vi "五参数标样核查.vi"(11 "启动参数":T1={"测量模式"="标样核查", "数据类型"="N", "输出参数"={"水温"=FALSE, "pH"=FALSE, "DO"=FALSE, "浊度"=FALSE, "电导率"=FALSE, "叶绿素a"=FALSE, "蓝绿藻"=FALSE, "藻密度"=FALSE, "ORP"=FALSE}}) -> ()   [LabVIEW 2016, in "斯坦道原位多参数.lvlib"]
panel:
  out "枚举":T2(ring)
  out "状态":string
  out "数值":i32
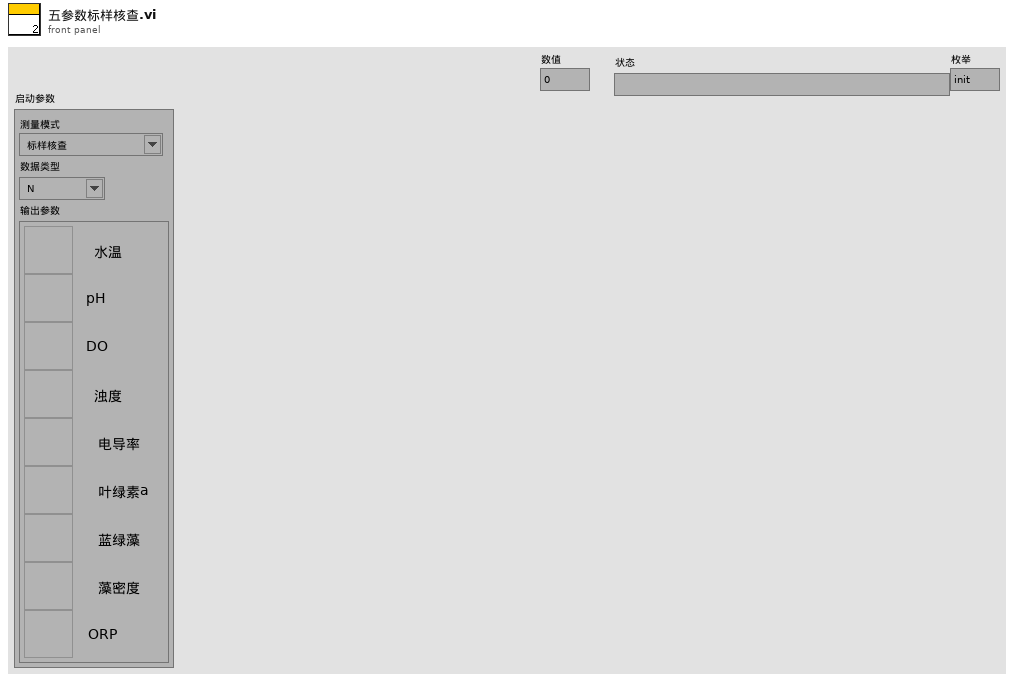
[diagram p1: front panel]
types:
  T1 = typedef "斯坦道原位多参数.lvlib/标样核查启动自定义输入参数.ctl" = cluster{"测量模式":string, "数据类型":string, "输出参数":cluster{"水温":bool, "pH":bool, "DO":bool, "浊度":bool, "电导率":bool, "叶绿素a":bool, "蓝绿藻":bool, "藻密度":bool, "ORP":bool}}
  T2 = enum16{"init", "开机", "启动测量", "读取测量值", "存储数据", "关闭测量", "关机", "结束"}
  T3 = cluster{"时间标识":timestamp, "设备":string, "日志信息":string, "流程参数":string}
  T4 = cluster{"系统时间":timestamp, "工作状态":u16, "测量模式":u16, "告警代码":enum16{"无告警", "缺试剂告警", "缺水样告警", "缺蒸馏水告警", "缺标液告警", "仪表漏液告警", "标定异常告警", "超量程告警", "加热异常", "低试剂预警", "超上限告警", "超下限告警", "仪表内部其他异常", "滴定异常告警", "电极异常告警", "量程切换告警", "参数设置告警", "PH电极电位异常", "电导率电极异常", "浊度光度异常", "溶解氧电极异常", "溶解氧光强异常", "温度异常告警", "PH异常告警", "溶解氧异常告警", "电导率异常告警", "浊度异常告警", "叶绿素异常告警", "藻密度异常告警", "蓝绿藻异常告警", "ORP异常告警", "氨氮异常告警", "清洁刷异常告警", "SD卡异常告警", "蓝牙异常告警", "Wifi异常告警", "流程异常告警"}, "故障代码":enum16{"无故障", "电机故障", "温度故障", "通讯故障", "滴定故障"}, "日志代码":u16, "软件版本":string}
  T5 = cluster{"水温标准液标准浓度":dbl, "酸碱度标准液标准浓度":dbl, "溶解氧标准液标准浓度":dbl, "电导率标准液标准浓度":dbl, "浊度标准液标准浓度":dbl, "叶绿素a标准液标准浓度":dbl, "蓝绿藻标准液标准浓度":dbl, "ORP标准液标准浓度":dbl, "藻密度标准液标准浓度":dbl}
  T6 = cluster{"因子编码":string, "单位":string, "标样参考值":sgl, "水样数据时间":timestamp, "水样实测值":sgl, "水样数据标识":string, "K":sgl, "B":sgl, "T":sgl, "H":sgl, "水深":sgl, "探头温度":sgl, "信号值":sgl}
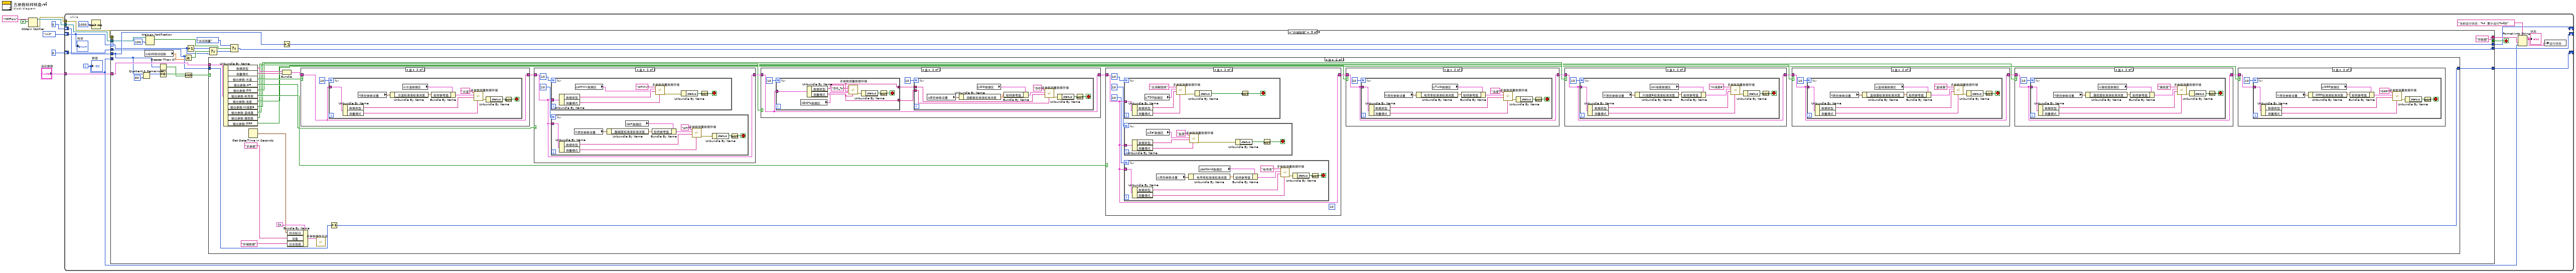
[diagram p0: block diagram]
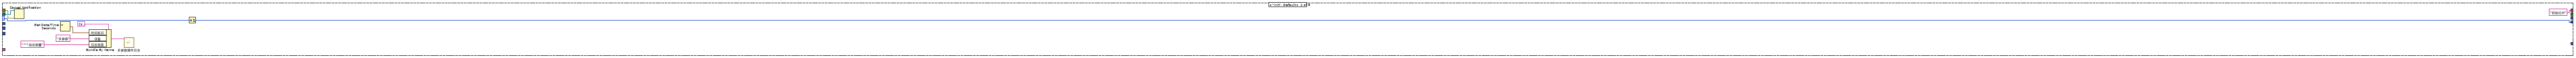
[diagram p2: hidden frame]
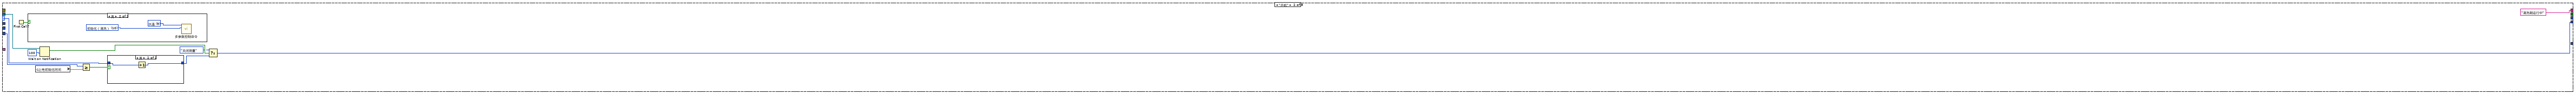
[diagram p3: hidden frame]
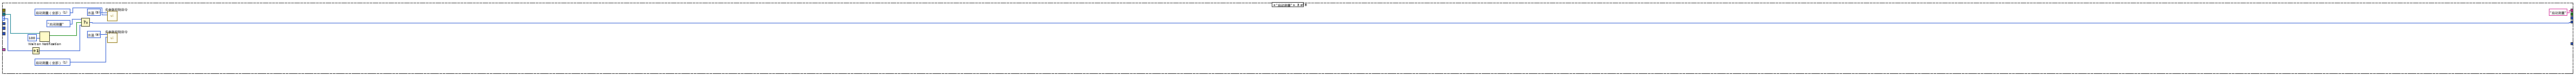
[diagram p6: hidden frame]
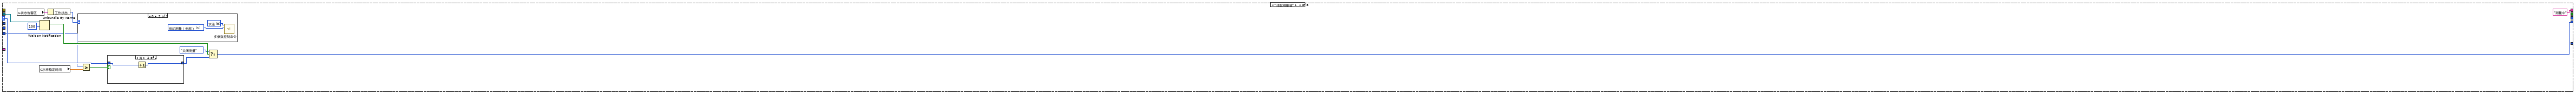
[diagram p7: hidden frame]
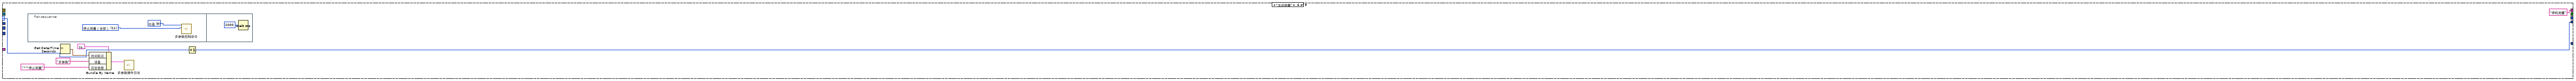
[diagram p20: hidden frame]
diagram:
  n1 = Obtain Notifier(name (unnamed)="MPFlow" ("名称（未命名）"), notification data type=FALSE) -> (notifier out=w5:refnum<notifier>, error out=w4:errorcluster)  [unwired: 2 in, 1 out]
  n2 = while {
    shift-right: [w19] -> _
    shift-left: T2."init" ("枚举") -> [w23]
    tunnel: w5 -> [w21]
    tunnel: w4 -> [w20]
    tunnel: "启动参数" -> [w13]
    shift-right: [w11] -> _
    shift-left: u32 0 ("等待时间（毫秒）") -> [w12]
    shift-right: [w9] -> _
    shift-left: u32 0 ("等待时间（毫秒）") -> [w10]
    i -> [w15]
    stop <- w22 stop-if-true
    n3 = Wait (ms)(milliseconds to wait=u32 1000 ("等待时间（毫秒）")) -> ()  [unwired: 1 out]
    n4 = case shown="\"存储数据\"" w23 {
      selector: w23 -> [w31 w45 w62 w75 w82 w300 w306 w310]
      tunnel: [_ _ _ _ _ _ _ TRUE] -> w22
      tunnel: w21 -> [w33 w41 w61 w72 w91 _ _ w307]
      tunnel: w20 -> [w32 _ _ _ _ _ _ _]
      tunnel: [w30 w39 w58 w70 w87 w299 w305 w309] -> w19
      tunnel: w15 -> [_ w44 _ w66 _ _ _ _]
      tunnel: ["初始化中" ("状态") "清洗刷运行中" ("状态") "启动测量" ("状态") "测量中" ("状态") "存数据" ("状态") "停机测量" ("状态") "关机" ("状态") "" ("状态")] -> w16
      tunnel: w13 -> [_ _ _ _ w100 _ _ _]
      tunnel: w12 -> [_ _ _ _ w94 _ _ _]
      tunnel: [_ _ _ _ w95 _ _ _] -> w11
      tunnel: w10 -> [_ _ _ _ w84 _ _ _]
      tunnel: [_ _ _ _ w86 _ _ _] -> w9
      frame "init", Default {
        n5 = Cancel Notification(0:w33, 3:w32) -> ()  [unwired: 3 out]
        n6 = Get Date/Time In Seconds() -> (seconds since 1Jan1904=w27:timestamp)
        n7 = Bundle By Name(cluster=T3 {"时间标识"=timestamp(0 s since 1904-01-01), "设备"="", "日志信息"="", "流程参数"=""} ("data in"), "时间标识"=w27, "设备"="多参数", "日志信息"="<<启动测量") -> (w26:T3)
        n8 = call "多参数操作日志.vi"("data"=w26) -> ()  [unwired: 10 in, 1 out]
        n9 = Increment(x=w31) -> (x+1=w30:T2)
      }
      frame "开机" {
        n10 = First Call?() -> (First Call?: T/F=w35:bool)
        n11 = case shown="真" w35 {
          frame False {
          }
          frame True {
            w47 = u16 10 items=["启动测量（全部）"=1, "初始化（清洗）"=10, "停止测量（全部）"=11, "校时"=13, "启动测量（单个传感器）"=19, "停止测量（单个传感器）"=20] ("控制命令")
            w46 = u16 9 items=["氨氮"=3, "水温"=9, "pH值"=10, "溶解氧"=11, "电导率"=12, "浊度"=13, "叶绿素a"=14, "藻密度"=15, "蓝绿藻"=16, "氧化还原电位"=17, "溶解氧%"=18, "盐度"=19] ("站号")
            n12 = call "多参数控制命令.vi"("控制命令"=w47, "站号"=w46) -> ()  [unwired: 9 in, 1 out]
          }
        }
        n13 = global read "多参数断电保存全局变量.vi" "上电初始化时间"() -> (w34:dbl)
        n14 = Wait on Notification(notifier=w41, timeout in ms (-1)=100 ("超时毫秒(-1)")) -> (notification=w42:bool)  [unwired: 2 in, 3 out]
        n15 = Greater Or Equal?(x=w44, y=w34) -> (x >= y?=w43:bool)
        n16 = case shown="真" w43 {
          tunnel: w45 -> [w48 w50]
          tunnel: [w48 w49] -> w40
          frame False {
          }
          frame True {
            n17 = Increment(x=w50) -> (x+1=w49:T2)
          }
        }
        n18 = Select(t=T2."关闭测量" ("枚举"), s=w42, f=w40) -> (s? t:f=w39:T2)
      }
      frame "启动测量" {
        w52 = u16 1 items=["启动测量（全部）"=1, "初始化（清洗）"=10, "停止测量（全部）"=11, "校时"=13, "启动测量（单个传感器）"=19, "停止测量（单个传感器）"=20] ("控制命令")
        w51 = u16 9 items=["氨氮"=3, "水温"=9, "pH值"=10, "溶解氧"=11, "电导率"=12, "浊度"=13, "叶绿素a"=14, "藻密度"=15, "蓝绿藻"=16, "氧化还原电位"=17, "溶解氧%"=18, "盐度"=19] ("站号")
        w53 = u16 1 items=["启动测量（全部）"=1, "初始化（清洗）"=10, "停止测量（全部）"=11, "校时"=13, "启动测量（单个传感器）"=19, "停止测量（单个传感器）"=20] ("控制命令")
        w54 = u16 9 items=["氨氮"=3, "水温"=9, "pH值"=10, "溶解氧"=11, "电导率"=12, "浊度"=13, "叶绿素a"=14, "藻密度"=15, "蓝绿藻"=16, "氧化还原电位"=17, "溶解氧%"=18, "盐度"=19] ("站号")
        n19 = Increment(x=w62) -> (x+1=w59:T2)
        n20 = Wait on Notification(notifier=w61, timeout in ms (-1)=100 ("超时毫秒(-1)")) -> (notification=w60:bool)  [unwired: 2 in, 3 out]
        n21 = Select(t=T2."关闭测量" ("枚举"), s=w60, f=w59) -> (s? t:f=w58:T2)
        n22 = call "多参数控制命令.vi"("控制命令"=w53, "站号"=w54) -> ()  [unwired: 9 in, 1 out]
        n23 = call "多参数控制命令.vi"("控制命令"=w52, "站号"=w51) -> ()  [unwired: 9 in, 1 out]
      }
      frame "读取测量值" {
        n24 = global read "多参数全局变量.vi" "状态告警区"() -> (w65:T4)
        n25 = global read "多参数断电保存全局变量.vi" "水样稳定时间"() -> (w63:dbl)
        n26 = Wait on Notification(notifier=w72, timeout in ms (-1)=100 ("超时毫秒(-1)")) -> (notification=w73:bool)  [unwired: 2 in, 3 out]
        n27 = Unbundle By Name(w65) -> ("工作状态"=w64:u16)
        n28 = case shown="0" w64 {
          frame Default {
          }
          frame 0 {
            w76 = u16 1 items=["启动测量（全部）"=1, "初始化（清洗）"=10, "停止测量（全部）"=11, "校时"=13, "启动测量（单个传感器）"=19, "停止测量（单个传感器）"=20] ("控制命令")
            w77 = u16 9 items=["氨氮"=3, "水温"=9, "pH值"=10, "溶解氧"=11, "电导率"=12, "浊度"=13, "叶绿素a"=14, "藻密度"=15, "蓝绿藻"=16, "氧化还原电位"=17, "溶解氧%"=18, "盐度"=19] ("站号")
            n29 = call "多参数控制命令.vi"("控制命令"=w76, "站号"=w77) -> ()  [unwired: 9 in, 1 out]
          }
        }
        n30 = Greater Or Equal?(x=w66, y=w63) -> (x >= y?=w74:bool)
        n31 = case shown="真" w74 {
          tunnel: w75 -> [w78 w80]
          tunnel: [w78 w79] -> w71
          frame False {
          }
          frame True {
            n32 = Increment(x=w80) -> (x+1=w79:T2)
          }
        }
        n33 = Select(t=T2."关闭测量" ("枚举"), s=w73, f=w71) -> (s? t:f=w70:T2)
      }
      frame "存储数据" {
        n34 = Quotient & Remainder(x=w94, y=u32 60) -> (x-y*floor(x/y)=w98:u32)  [unwired: 1 out]
        n35 = global read "多参数断电保存全局变量.vi" "标样测试组数"() -> (w81:dbl)
        n36 = Wait on Notification(notifier=w91, timeout in ms (-1)=100 ("超时毫秒(-1)")) -> (notification=w90:bool)  [unwired: 2 in, 3 out]
        n37 = Greater Than 0?(x=w94) -> (x > 0?=w93:bool)
        n38 = Equal To 0?(x=w98) -> (x = 0?=w97:bool)
        n39 = Greater Or Equal?(x=w84, y=w81) -> (x >= y?=w85:bool)
        n40 = Compound Arithmetic op=AND ("复合运算")(w97, w93) -> (w96:bool)
        n41 = Increment(x=w82) -> (x+1=w83:T2)
        n42 = Select(t=w83, s=w85, f=w82) -> (s? t:f=w89:T2)
        n43 = case shown="真" w96 {
          tunnel: w100 -> [_ w130]
          tunnel: w84 -> [w102 w112]
          tunnel: [w102 w111] -> w86
          frame False {
          }
          frame True {
            n44 = Unbundle By Name(w130) -> ("数据类型"=w129:string, "测量模式"=w128:string, "输出参数.水温"=w117:bool, "输出参数.pH"=w116:bool, "输出参数.DO"=w115:bool, "输出参数.电导率"=w114:bool, "输出参数.浊度"=w113:bool, "输出参数.叶绿素a"=w106:bool, "输出参数.蓝绿藻"=w105:bool, "输出参数.藻密度"=w104:bool, "输出参数.ORP"=w103:bool)
            n45 = Get Date/Time In Seconds() -> (seconds since 1Jan1904=w121:timestamp)
            n46 = Bundle("数据类型"=w129, "测量模式"=w128) -> (w127:cluster{"数据类型":string, "测量模式":string})  [unwired: 1 in]
            n47 = Bundle By Name(cluster=T3 {"时间标识"=timestamp(0 s since 1904-01-01), "设备"="", "日志信息"="", "流程参数"=""} ("data in"), "时间标识"=w121, "设备"="多参数", "日志信息"="存储数据") -> (w120:T3)
            n48 = case shown="真" w117 {
              tunnel: w127 -> [w279 w281]
              tunnel: [w279 w281] -> w126
              frame False {
              }
              frame True {
                n49 = for {
                  N: 10 -> [_]
                  tunnel: w281 -> [w292]
                  stop <- w286 stop-if-true
                  n50 = Unbundle By Name(w292) -> ("数据类型"=w283:string, "测量模式"=w282:string)
                  n51 = global read "多参数断电保存全局变量.vi" "质控参数设置"() -> (w290:T5)
                  n52 = Unbundle By Name(w290) -> ("水温标准液标准浓度"=w289:dbl)
                  n53 = global read "多参数全局变量.vi" "水温数据区"() -> (w291:T6)
                  n54 = Bundle By Name(cluster=w291, "标样参考值"=w289) -> (w285:T6)
                  n55 = call "多参数测量数据存储.vi"("测量模式"=w282, "数据类型"=w283, "数据区"=w285, "table输入"="水温") -> ("error out"=w288:errorcluster)  [unwired: 7 in]
                  n56 = Unbundle By Name(w288) -> ("status"=w287:bool)
                  n57 = Not(x=w287) -> (.not. x?=w286:bool)
                }
              }
            }
            n58 = call "多参数操作日志.vi"("data"=w120) -> ()  [unwired: 10 in, 1 out]
            n59 = Increment(x=w112) -> (x+1=w111:u32)
            n60 = case shown="真" w116 {
              tunnel: w126 -> [w256 w259]
              tunnel: [w256 w259] -> w124
              frame False {
              }
              frame True {
                n61 = for {
                  N: 10 -> [_]
                  tunnel: w259 -> [w267]
                  stop <- w264 stop-if-true
                  n62 = Unbundle By Name(w267) -> ("数据类型"=w261:string, "测量模式"=w260:string)
                  n63 = global read "多参数全局变量.vi" "pHmv数据区"() -> (w262:T6)
                  n64 = call "多参数测量数据存储.vi"("测量模式"=w260, "数据类型"=w261, "数据区"=w262, "table输入"="pHmv") -> ("error out"=w266:errorcluster)  [unwired: 7 in]
                  n65 = Unbundle By Name(w266) -> ("status"=w265:bool)
                  n66 = Not(x=w265) -> (.not. x?=w264:bool)
                }
                n67 = for {
                  N: 10 -> [_]
                  tunnel: w259 -> [w278]
                  stop <- w272 stop-if-true
                  n68 = Unbundle By Name(w278) -> ("数据类型"=w269:string, "测量模式"=w268:string)
                  n69 = global read "多参数断电保存全局变量.vi" "质控参数设置"() -> (w277:T5)
                  n70 = Unbundle By Name(w277) -> ("酸碱度标准液标准浓度"=w276:dbl)
                  n71 = global read "多参数全局变量.vi" "pH数据区"() -> (w275:T6)
                  n72 = Bundle By Name(cluster=w275, "标样参考值"=w276) -> (w270:T6)
                  n73 = call "多参数测量数据存储.vi"("测量模式"=w268, "数据类型"=w269, "数据区"=w270, "table输入"="pH") -> ("error out"=w274:errorcluster)  [unwired: 7 in]
                  n74 = Unbundle By Name(w274) -> ("status"=w273:bool)
                  n75 = Not(x=w273) -> (.not. x?=w272:bool)
                }
              }
            }
            n76 = case shown="真" w115 {
              tunnel: [w232 w237] -> w125
              tunnel: w124 -> [w232 w237]
              frame False {
              }
              frame True {
                n77 = for {
                  N: 10 -> [_]
                  tunnel: w237 -> [w255]
                  tunnel: [w249] -> w236
                  tunnel: [w248] -> w235
                  stop <- w252 stop-if-true
                  n78 = global read "多参数全局变量.vi" "DO%数据区"() -> (w250:T6)
                  n79 = Unbundle By Name(w255) -> ("数据类型"=w248:string, "测量模式"=w249:string)
                  n80 = call "多参数测量数据存储.vi"("测量模式"=w249, "数据类型"=w248, "数据区"=w250, "table输入"="DO_%") -> ("error out"=w254:errorcluster)  [unwired: 7 in]
                  n81 = Unbundle By Name(w254) -> ("status"=w253:bool)
                  n82 = Not(x=w253) -> (.not. x?=w252:bool)
                }
                n83 = for {
                  N: 10 -> [_]
                  tunnel: w236 -> [w238]
                  tunnel: w235 -> [w241]
                  stop <- w242 stop-if-true
                  n84 = global read "多参数断电保存全局变量.vi" "质控参数设置"() -> (w247:T5)
                  n85 = Unbundle By Name(w247) -> ("溶解氧标准液标准浓度"=w246:dbl)
                  n86 = global read "多参数全局变量.vi" "DO数据区"() -> (w245:T6)
                  n87 = Bundle By Name(cluster=w245, "标样参考值"=w246) -> (w239:T6)
                  n88 = call "多参数测量数据存储.vi"("测量模式"=w238, "数据类型"=w241, "数据区"=w239, "table输入"="DO") -> ("error out"=w244:errorcluster)  [unwired: 7 in]
                  n89 = Unbundle By Name(w244) -> ("status"=w243:bool)
                  n90 = Not(x=w243) -> (.not. x?=w242:bool)
                }
              }
            }
            n91 = case shown="真" w114 {
              tunnel: w125 -> [w200 w204]
              tunnel: [w200 w204] -> w123
              frame False {
              }
              frame True {
                (unwired) 10
                n92 = for {
                  N: 10 -> [_]
                  tunnel: w204 -> [w212]
                  stop <- w209 stop-if-true
                  n93 = Unbundle By Name(w212) -> ("数据类型"=w206:string, "测量模式"=w205:string)
                  n94 = global read "多参数全局变量.vi" "TDS数据区"() -> (w207:T6)
                  n95 = call "多参数测量数据存储.vi"("测量模式"=w205, "数据类型"=w206, "数据区"=w207, "table输入"="总溶解固体") -> ("error out"=w211:errorcluster)  [unwired: 7 in]
                  n96 = Unbundle By Name(w211) -> ("status"=w210:bool)
                  n97 = Not(x=w210) -> (.not. x?=w209:bool)
                }
                n98 = for {
                  N: 10 -> [_]
                  tunnel: w204 -> [w231]
                  stop <- w228 stop-if-true
                  n99 = Unbundle By Name(w231) -> ("数据类型"=w225:string, "测量模式"=w224:string)
                  n100 = global read "多参数全局变量.vi" "Sal数据区"() -> (w226:T6)
                  n101 = call "多参数测量数据存储.vi"("测量模式"=w224, "数据类型"=w225, "数据区"=w226, "table输入"="盐度") -> ("error out"=w230:errorcluster)  [unwired: 7 in]
                  n102 = Unbundle By Name(w230) -> ("status"=w229:bool)
                  n103 = Not(x=w229) -> (.not. x?=w228:bool)
                }
                n104 = for {
                  N: 10 -> [_]
                  tunnel: w204 -> [w223]
                  stop <- w217 stop-if-true
                  n105 = Unbundle By Name(w223) -> ("数据类型"=w214:string, "测量模式"=w213:string)
                  n106 = global read "多参数断电保存全局变量.vi" "质控参数设置"() -> (w222:T5)
                  n107 = Unbundle By Name(w222) -> ("电导率标准液标准浓度"=w221:dbl)
                  n108 = global read "多参数全局变量.vi" "spCond数据区"() -> (w220:T6)
                  n109 = Bundle By Name(cluster=w220, "标样参考值"=w221) -> (w215:T6)
                  n110 = call "多参数测量数据存储.vi"("测量模式"=w213, "数据类型"=w214, "数据区"=w215, "table输入"="电导率") -> ("error out"=w219:errorcluster)  [unwired: 7 in]
                  n111 = Unbundle By Name(w219) -> ("status"=w218:bool)
                  n112 = Not(x=w218) -> (.not. x?=w217:bool)
                }
              }
            }
            n113 = case shown="真" w113 {
              tunnel: w123 -> [w186 w187]
              tunnel: [w186 w187] -> w109
              frame False {
              }
              frame True {
                n114 = for {
                  N: 10 -> [_]
                  tunnel: w187 -> [w199]
                  stop <- w193 stop-if-true
                  n115 = Unbundle By Name(w199) -> ("数据类型"=w190:string, "测量模式"=w189:string)
                  n116 = global read "多参数断电保存全局变量.vi" "质控参数设置"() -> (w198:T5)
                  n117 = Unbundle By Name(w198) -> ("电导率标准液标准浓度"=w197:dbl)
                  n118 = global read "多参数全局变量.vi" "Turb数据区"() -> (w196:T6)
                  n119 = Bundle By Name(cluster=w196, "标样参考值"=w197) -> (w191:T6)
                  n120 = call "多参数测量数据存储.vi"("测量模式"=w189, "数据类型"=w190, "数据区"=w191, "table输入"="浊度") -> ("error out"=w195:errorcluster)  [unwired: 7 in]
                  n121 = Unbundle By Name(w195) -> ("status"=w194:bool)
                  n122 = Not(x=w194) -> (.not. x?=w193:bool)
                }
              }
            }
            n123 = case shown="真" w106 {
              tunnel: w109 -> [w172 w173]
              tunnel: [w172 w173] -> w110
              frame False {
              }
              frame True {
                n124 = for {
                  N: 10 -> [_]
                  tunnel: w173 -> [w185]
                  stop <- w179 stop-if-true
                  n125 = Unbundle By Name(w185) -> ("数据类型"=w176:string, "测量模式"=w175:string)
                  n126 = global read "多参数断电保存全局变量.vi" "质控参数设置"() -> (w184:T5)
                  n127 = Unbundle By Name(w184) -> ("叶绿素a标准液标准浓度"=w183:dbl)
                  n128 = global read "多参数全局变量.vi" "叶绿素数据区"() -> (w182:T6)
                  n129 = Bundle By Name(cluster=w182, "标样参考值"=w183) -> (w177:T6)
                  n130 = call "多参数测量数据存储.vi"("测量模式"=w175, "数据类型"=w176, "数据区"=w177, "table输入"="叶绿素a") -> ("error out"=w181:errorcluster)  [unwired: 7 in]
                  n131 = Unbundle By Name(w181) -> ("status"=w180:bool)
                  n132 = Not(x=w180) -> (.not. x?=w179:bool)
                }
              }
            }
            n133 = case shown="真" w105 {
              tunnel: w110 -> [w158 w159]
              tunnel: [w158 w159] -> w108
              frame False {
              }
              frame True {
                n134 = for {
                  N: 10 -> [_]
                  tunnel: w159 -> [w171]
                  stop <- w165 stop-if-true
                  n135 = Unbundle By Name(w171) -> ("数据类型"=w162:string, "测量模式"=w161:string)
                  n136 = global read "多参数断电保存全局变量.vi" "质控参数设置"() -> (w170:T5)
                  n137 = Unbundle By Name(w170) -> ("蓝绿藻标准液标准浓度"=w169:dbl)
                  n138 = global read "多参数全局变量.vi" "蓝绿藻数据区"() -> (w168:T6)
                  n139 = Bundle By Name(cluster=w168, "标样参考值"=w169) -> (w163:T6)
                  n140 = call "多参数测量数据存储.vi"("测量模式"=w161, "数据类型"=w162, "数据区"=w163, "table输入"="蓝绿藻") -> ("error out"=w167:errorcluster)  [unwired: 7 in]
                  n141 = Unbundle By Name(w167) -> ("status"=w166:bool)
                  n142 = Not(x=w166) -> (.not. x?=w165:bool)
                }
              }
            }
            n143 = case shown="真" w104 {
              tunnel: w108 -> [w144 w145]
              tunnel: [w144 w145] -> w107
              frame False {
              }
              frame True {
                n144 = for {
                  N: 10 -> [_]
                  tunnel: w145 -> [w157]
                  stop <- w151 stop-if-true
                  n145 = Unbundle By Name(w157) -> ("数据类型"=w148:string, "测量模式"=w147:string)
                  n146 = global read "多参数断电保存全局变量.vi" "质控参数设置"() -> (w156:T5)
                  n147 = Unbundle By Name(w156) -> ("藻密度标准液标准浓度"=w155:dbl)
                  n148 = global read "多参数全局变量.vi" "藻密度数据区"() -> (w154:T6)
                  n149 = Bundle By Name(cluster=w154, "标样参考值"=w155) -> (w149:T6)
                  n150 = call "多参数测量数据存储.vi"("测量模式"=w147, "数据类型"=w148, "数据区"=w149, "table输入"="藻密度") -> ("error out"=w153:errorcluster)  [unwired: 7 in]
                  n151 = Unbundle By Name(w153) -> ("status"=w152:bool)
                  n152 = Not(x=w152) -> (.not. x?=w151:bool)
                }
              }
            }
            n153 = case shown="真" w103 {
              tunnel: w107 -> [_ w132]
              frame False {
              }
              frame True {
                n154 = for {
                  N: 10 -> [_]
                  tunnel: w132 -> [w143]
                  stop <- w137 stop-if-true
                  n155 = Unbundle By Name(w143) -> ("数据类型"=w134:string, "测量模式"=w133:string)
                  n156 = global read "多参数断电保存全局变量.vi" "质控参数设置"() -> (w142:T5)
                  n157 = Unbundle By Name(w142) -> ("ORP标准液标准浓度"=w141:dbl)
                  n158 = global read "多参数全局变量.vi" "ORP数据区"() -> (w140:T6)
                  n159 = Bundle By Name(cluster=w140, "标样参考值"=w141) -> (w135:T6)
                  n160 = call "多参数测量数据存储.vi"("测量模式"=w133, "数据类型"=w134, "数据区"=w135, "table输入"="ORP") -> ("error out"=w139:errorcluster)  [unwired: 7 in]
                  n161 = Unbundle By Name(w139) -> ("status"=w138:bool)
                  n162 = Not(x=w138) -> (.not. x?=w137:bool)
                }
              }
            }
          }
        }
        n163 = Select(t=T2."关闭测量", s=w90, f=w89) -> (s? t:f=w87:T2)
        n164 = Increment(x=w94) -> (x+1=w95:u32)
      }
      frame "关闭测量" {
        n165 = flat-sequence {
          frame #0 {
            w301 = u16 11 items=["启动测量（全部）"=1, "初始化（清洗）"=10, "停止测量（全部）"=11, "校时"=13, "启动测量（单个传感器）"=19, "停止测量（单个传感器）"=20] ("控制命令")
            w302 = u16 9 items=["氨氮"=3, "水温"=9, "pH值"=10, "溶解氧"=11, "电导率"=12, "浊度"=13, "叶绿素a"=14, "藻密度"=15, "蓝绿藻"=16, "氧化还原电位"=17, "溶解氧%"=18, "盐度"=19] ("站号")
            n166 = call "多参数控制命令.vi"("控制命令"=w301, "站号"=w302) -> ()  [unwired: 9 in, 1 out]
          }
          frame #1 {
            n167 = Wait (ms)(milliseconds to wait=u32 2000 ("等待时间（毫秒）")) -> ()  [unwired: 1 out]
          }
        }
        n168 = Get Date/Time In Seconds() -> (seconds since 1Jan1904=w296:timestamp)
        n169 = Bundle By Name(cluster=T3 {"时间标识"=timestamp(0 s since 1904-01-01), "设备"="", "日志信息"="", "流程参数"=""} ("data in"), "时间标识"=w296, "设备"="多参数", "日志信息"=">>停止测量") -> (w295:T3)
        n170 = call "多参数操作日志.vi"("data"=w295) -> ()  [unwired: 10 in, 1 out]
        n171 = Increment(x=w300) -> (x+1=w299:T2)
      }
      frame "关机" {
        n172 = Increment(x=w306) -> (x+1=w305:T2)
      }
      frame "结束" {
        n173 = Release Notifier(notifier=w307) -> ()  [unwired: 2 in, 3 out]
        n174 = Increment(x=w310) -> (x+1=w309:T2)
      }
    }
    n175 = Format Into String(format string="当前运行状态：%s  累计运行%d秒" ("格式字符串"), w16, w15) -> (resulting string=w14:string)  [unwired: 2 in, 1 out]
    "状态" <- w14
    n176 = global write "多参数全局变量.vi" "运行状态"(w14) -> ()
    "数值" <- w15
    "枚举" <- w23
  }
